vi "TDMS Header Writer.vi"(9 "Data Cluster":T1 {"Amplifier Model" items=["Select a Model", "AM 1700", "BMA 200"]}, 11 "tdms file":refnum<k34>) -> (1 "Start Time hr/min":string, 2 "Date mm/dd/yy":string, 3 "tdms file out":refnum<k34>)   [LabVIEW 2014]
panel:
  # "Inputs"
  # "Outputs"
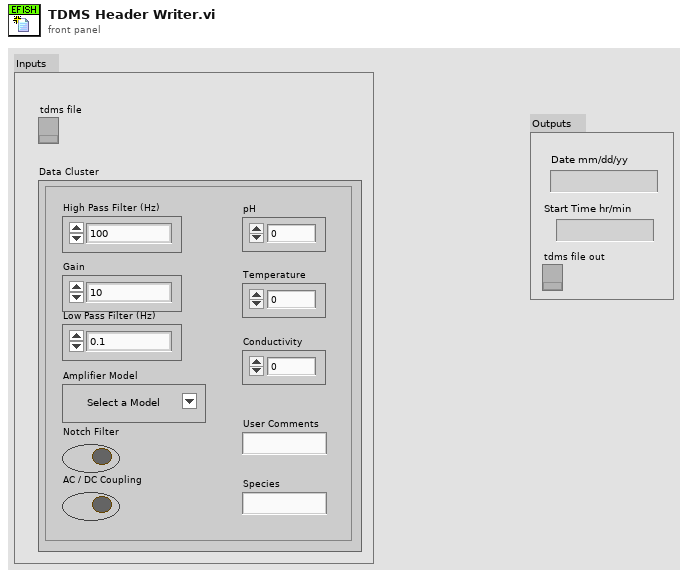
[diagram p1: front panel]
types:
  T1 = cluster{"High Pass Filter (Hz)":enum16{"100", "500", "1000", "3000", "5000", "10,000", "20,000", "30,000", "50,000"}, "Gain":enum16{"10", "20", "50", "100", "200", "500", "1000", "2k", "5k", "10k", "20k", "50k"}, "Low Pass Filter (Hz)":enum16{"0.1", "1", "3", "10", "30", "100", "300"}, "Amplifier Model":u16, "Notch Filter":bool, "AC / DC Coupling":bool, "Temperature":dbl, "Conductivity":dbl, "pH":dbl, "User Comments":string, "Species":string}
  T2 = enum16{"100", "500", "1000", "3000", "5000", "10,000", "20,000", "30,000", "50,000"}
  T3 = enum16{"10", "20", "50", "100", "200", "500", "1000", "2k", "5k", "10k", "20k", "50k"}
  T4 = enum16{"0.1", "1", "3", "10", "30", "100", "300"}
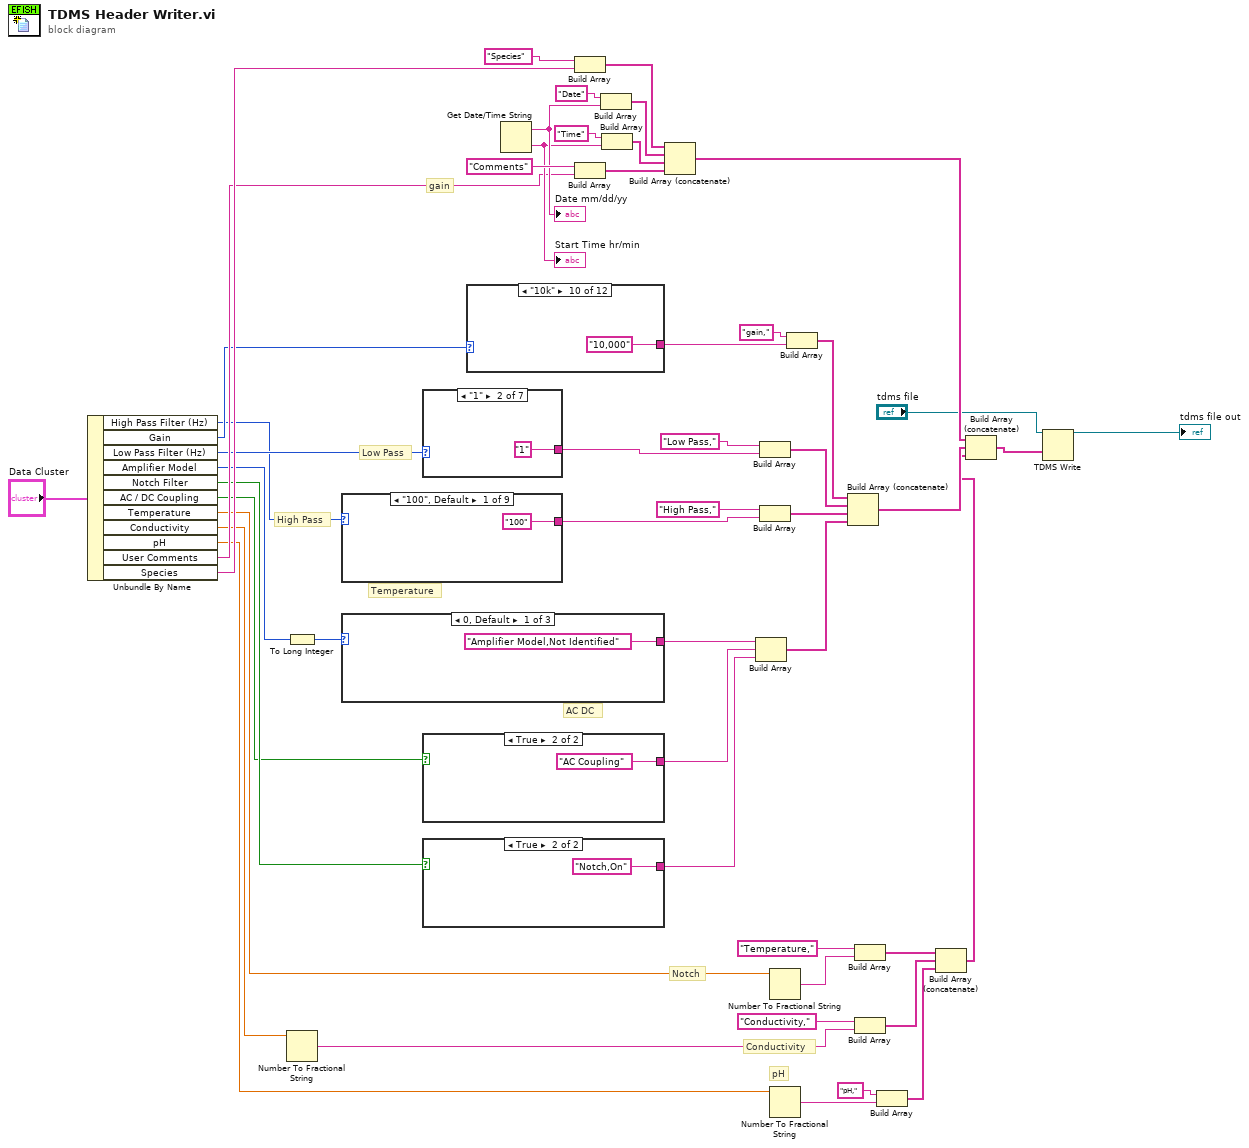
[diagram p0: block diagram]
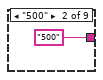
[diagram p2: hidden frame]
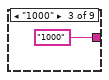
[diagram p3: hidden frame]
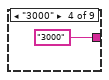
[diagram p4: hidden frame]
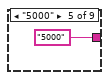
[diagram p5: hidden frame]
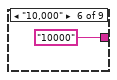
[diagram p6: hidden frame]
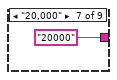
[diagram p7: hidden frame]
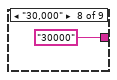
[diagram p8: hidden frame]
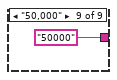
[diagram p9: hidden frame]
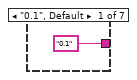
[diagram p10: hidden frame]
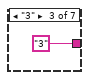
[diagram p11: hidden frame]
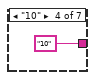
[diagram p12: hidden frame]
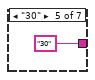
[diagram p13: hidden frame]
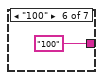
[diagram p14: hidden frame]
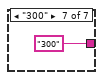
[diagram p15: hidden frame]
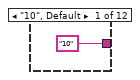
[diagram p16: hidden frame]
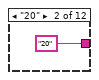
[diagram p17: hidden frame]
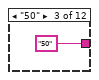
[diagram p18: hidden frame]
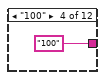
[diagram p19: hidden frame]
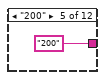
[diagram p20: hidden frame]
diagram:
  # "Low Pass"
  # "pH"
  # "Conductivity"
  # "Temperature"
  # "High Pass"
  # "Notch"
  # "AC DC"
  # "gain"
  n1 = Unbundle By Name("Data Cluster") -> ("High Pass Filter (Hz)"=w8:T2, "Gain"=w11:T3, "Low Pass Filter (Hz)"=w10:T4, "Amplifier Model"=w14:u16, "Notch Filter"=w17:bool, "AC / DC Coupling"=w16:bool, "Temperature"=w18:dbl, "Conductivity"=w19:dbl, "pH"=w20:dbl, "User Comments"=w21:string, "Species"=w22:string)
  n2 = To Long Integer(number=w14) -> (32bit integer=w15:i32)
  n3 = Number To Fractional String(number=w19) -> (F-format string=w28:string)  [unwired: 3 in]
  n4 = case shown="\"100\", Default" w8 {
    tunnel: ["100" "500" "1000" "3000" "5000" "10000" "20000" "30000" "50000"] -> w7
    frame "100", Default {
    }
    frame "500" {
    }
    frame "1000" {
    }
    frame "3000" {
    }
    frame "5000" {
    }
    frame "10,000" {
    }
    frame "20,000" {
    }
    frame "30,000" {
    }
    frame "50,000" {
    }
  }
  n5 = case shown="0, Default" w15 {
    tunnel: ["Amplifier Model,Not Identified" "Model,AM 1700" "Amplify Model,BMA 200"] -> w13
    frame 0, Default {
    }
    frame 1 {
    }
    frame 2 {
    }
  }
  n6 = case shown="\"1\"" w10 {
    tunnel: ["0.1" "1" "3" "10" "30" "100" "300"] -> w9
    frame "0.1", Default {
    }
    frame "1" {
    }
    frame "3" {
    }
    frame "10" {
    }
    frame "30" {
    }
    frame "100" {
    }
    frame "300" {
    }
  }
  n7 = case shown="True" w16 {
    tunnel: ["DC Coupling" "AC Coupling"] -> w33
    frame False {
    }
    frame True {
    }
  }
  n8 = case shown="True" w17 {
    tunnel: ["Notch,Off" "Notch,On"] -> w32
    frame False {
    }
    frame True {
    }
  }
  n9 = case shown="\"10k\"" w11 {
    tunnel: ["10" "20" "50" "100" "200" "500" "1000" "2000" "5000" "10,000" "20,000" "50,000"] -> w12
    frame "10", Default {
    }
    frame "20" {
    }
    frame "50" {
    }
    frame "100" {
    }
    frame "200" {
    }
    frame "500" {
    }
    frame "1000" {
    }
    frame "2k" {
    }
    frame "5k" {
    }
    frame "10k" {
    }
    frame "20k" {
    }
    frame "50k" {
    }
  }
  n10 = Get Date/Time String() -> (date string=w42:string, time string=w41:string)  [unwired: 3 in]
  "Date mm/dd/yy" <- w42
  "Start Time hr/min" <- w41
  n11 = Build Array("Species" ("element"), w22) -> (w46:string[])
  n12 = Build Array("Comments" ("element"), w21) -> (w43:string[])
  n13 = Build Array("Date" ("element"), w42) -> (w45:string[])
  n14 = Build Array("Time" ("element"), w41) -> (w44:string[])
  n15 = Build Array (concatenate)(w46, w45, w44, w43) -> (w6:string[])
  n16 = Build Array(w13, w33, w32) -> (w31:string[])
  n17 = Build Array("Low Pass," ("string"), w9) -> (w35:string[])
  n18 = Build Array("High Pass," ("string"), w7) -> (w34:string[])
  n19 = Number To Fractional String(number=w18) -> (F-format string=w30:string)  [unwired: 3 in]
  n20 = Number To Fractional String(number=w20) -> (F-format string=w25:string)  [unwired: 3 in]
  n21 = Build Array("gain," ("string"), w12) -> (w36:string[])
  n22 = Build Array (concatenate)(w36, w35, w34, w31) -> (w5:string[])
  n23 = Build Array("Temperature," ("string"), w30) -> (w27:string[])
  n24 = Build Array("Conductivity," ("string"), w28) -> (w26:string[])
  n25 = Build Array("pH," ("element"), w25) -> (w23:string[])
  n26 = Build Array (concatenate)(w27, w26, w23) -> (w4:string[])
  n27 = Build Array (concatenate)(w6, w5, w4) -> (w3:string[])
  n28 = TDMS Write(0:"tdms file", 9:w3) -> (4:→"tdms file out":refnum<k34>)  [unwired: 4 in, 3 out]
